vi "WaitOnFinalProcessSync.vi"(8 "error in (no error)":errorcluster, 9 "timeout in ms (-1)":i32=-1, 11 "SMO":refnum<class "SMO.lvclass">) -> (0 "error out":errorcluster, 3 "SMO out":refnum<class "SMO.lvclass">)   [LabVIEW 2019, in "SMO.lvclass"]
doc: "This method is used to synchronize processes during launch and shutdown\n\nNote: This method is overridable by descendant\n\n---------------------------------------------------------------\nJKI State Machine Objects™\nhttp://jki.net/state-machine-objects/\nCopyright (C) 2005-2015, JKI <info@jki.net>\nALL RIGHTS RESERVEDJKI State Machine Objects (SMO) 1.3.0.56\nJKI - JKI\nCopyright (c) 2017, JKI"
uses:
  SMO.lvclass
panel:
  # "For instructions on how to use the JKI State Machine Objects, examples and video tutorials, visit:\nhttp://jki.net/state-machine-objects/\n\nJKI State Machine Objects™\nhttp://jki.net/state-machine-objects/\nCopyright (C) 2005-2015, JKI <info@jki.net>\nALL RIGHTS RESERVED"
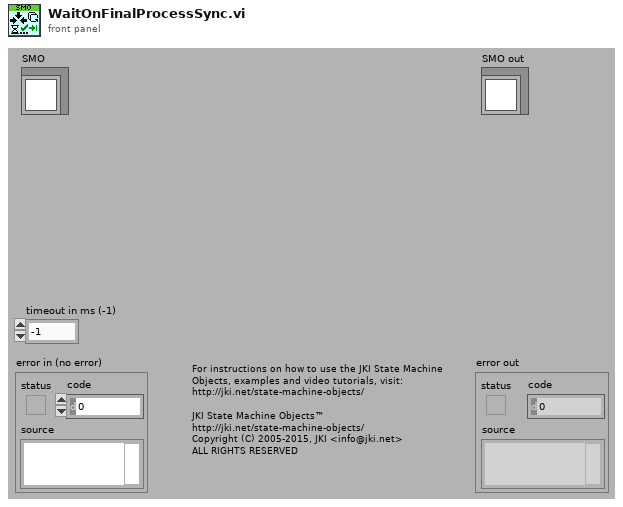
[diagram p1: front panel]
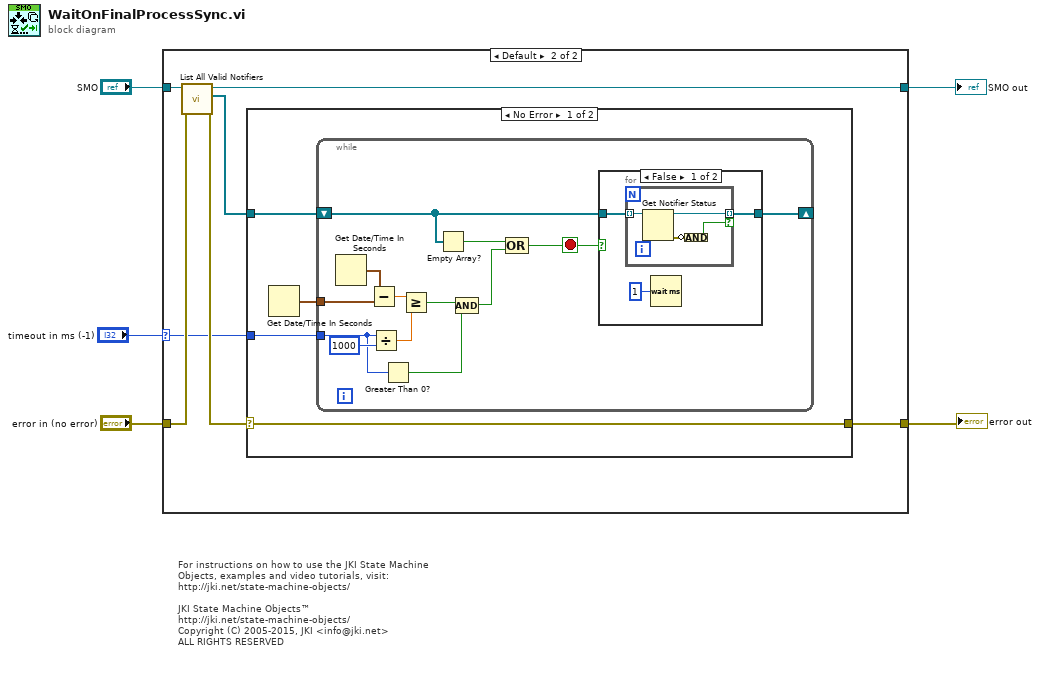
[diagram p0: block diagram]
diagram:
  # "For instructions on how to use the JKI State Machine Objects, examples and video tutorials, visit:\nhttp://jki.net/state-machine-objects/\n\nJKI State Machine Objects™\nhttp://jki.net/state-machine-objects/\nCopyright (C) 2005-2015, JKI <info@jki.net>\nALL RIGHTS RESERVED"
  n1 = case shown="Default" "timeout in ms (-1)" {
    selector: "timeout in ms (-1)" -> [_ w8]
    tunnel: "error in (no error)" -> [w6 w14]
    tunnel: [w6 w13] -> w4
    tunnel: [w7 w12] -> w3
    tunnel: "SMO" -> [w7 w11]
    frame 0 {
      # "Do not wait"
    }
    frame Default {
      n2 = call "List All Valid Notifiers.vi"("error in (no error)"=w14, "SMO"=w11) -> ("error out"=w9:errorcluster, "Valid Notifiers"=w10:refnum<notifier>[], "SMO out"=w12:refnum<class "SMO.lvclass">)  [unwired: 7 in]
      n3 = case shown="No Error" w9 {
        selector: w9 -> [w17 w40]
        tunnel: w10 -> [w18 _]
        tunnel: [w17 w40] -> w13
        tunnel: w8 -> [w16 _]
        frame No Error {
          n4 = Get Date/Time In Seconds() -> (seconds since 1Jan1904=w15:timestamp)
          n5 = while {
            shift-right: [w30] -> _
            shift-left: w18 -> [w31]
            tunnel: w16 -> [w23]
            tunnel: w15 -> [w28]
            stop <- w19 stop-if-true
            n6 = Get Date/Time In Seconds() -> (seconds since 1Jan1904=w29:timestamp)
            n7 = Subtract(x=w29, y=w28) -> (x-y=w27:dbl)
            n8 = Divide(x=w23, y=1000) -> (x/y=w25:dbl)
            n9 = Greater Than 0?(x=w23) -> (x > 0?=w22:bool)
            n10 = Greater Or Equal?(x=w27, y=w25) -> (x >= y?=w24:bool)
            n11 = Empty Array?(array=w31) -> (empty?=w20:bool)
            n12 = Compound Arithmetic op=AND(w24, w22) -> (w21:bool)
            n13 = Compound Arithmetic op=OR(w20, w21) -> (w19:bool)
            n14 = case shown="False" w19 {
              tunnel: w31 -> [w34 w39]
              tunnel: [w33 w39] -> w30
              frame False {
                n15 = for {
                  tunnel: w34 -> [w38] mode=indexing
                  tunnel: [w37] -> w33 mode=indexing if=w35
                  n16 = Get Notifier Status(notifier=w38) -> (notifier out=w37:refnum<notifier>, error out=w36:errorcluster)  [unwired: 1 in, 3 out]
                  n17 = Compound Arithmetic op=AND(invert w36) -> (w35:bool)
                }
                n18 = Wait (ms)(milliseconds to wait=u32 1) -> ()  [unwired: 1 out]
              }
              frame True {
              }
            }
          }
        }
        frame Error {
        }
      }
    }
  }
  "error out" <- w4
  "SMO out" <- w3
